vi "TDMS delete channel.vi"(8 "error in (no error)":errorcluster, 9 "Channels":string[](array[string]), 10 "group name":string="Untitled", 11 "file path":path) -> (0 "error out":errorcluster, 1 "Deleted channels":string[](array[string]), 3 "file path out":path)   [LabVIEW 2016]
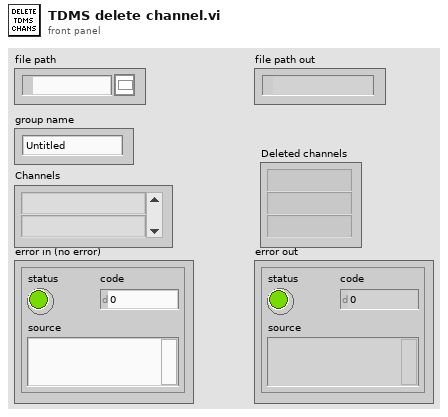
[diagram p1: front panel]
types:
  T1 = enum16{"open", "open or create", "create or replace", "create", "open (read-only)"}
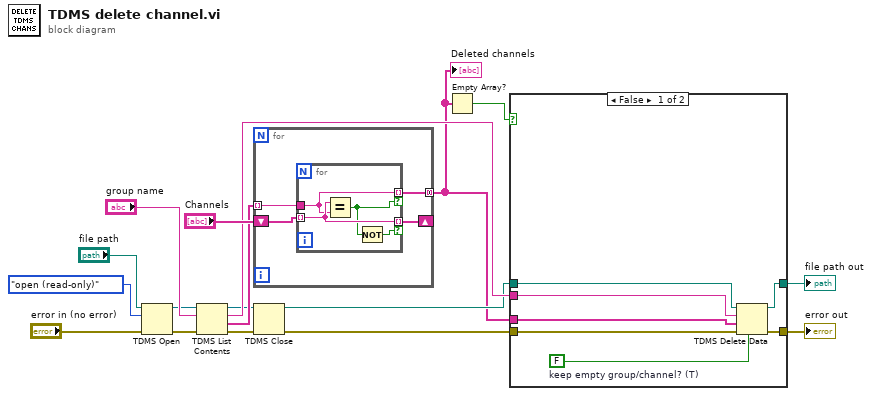
[diagram p0: block diagram]
diagram:
  n1 = TDMS Open(8:"error in (no error)", 10:T1."open (read-only)" ("operation (0:open)"), 11:"file path") -> (0:w13:errorcluster, 3:w16:refnum<k34>)  [unwired: 4 in]
  n2 = TDMS List Contents(4:w13, 6:"group name", 7:w16) -> (0:w9:errorcluster, 1:w11:string[], 2:w10:string, 3:w8:refnum<k34>)
  n3 = for {
    tunnel: w11 -> [w20] mode=indexing
    shift-right: [w19] -> _
    shift-left: "Channels" -> [w21]
    tunnel: [w18] -> w2 mode=concatenating
    n4 = for {
      tunnel: w21 -> [w25] mode=indexing
      tunnel: w20 -> [w23]
      tunnel: [w25] -> w19 mode=indexing if=w24
      tunnel: [w23] -> w18 mode=indexing if=w22
      n5 = Equal?(x=w25, y=w23) -> (x = y?=w22:bool)
      n6 = Not(x=w22) -> (.not. x?=w24:bool)
    }
  }
  "Deleted channels" <- w2
  n7 = TDMS Close(8:w9, 11:w8) -> (0:w5:errorcluster, 3:w6:path)
  n8 = Empty Array?(array=w2) -> (empty?=w1:bool)
  n9 = case shown="False" w1 {
    tunnel: w2 -> [w32 _]
    tunnel: w10 -> [w31 _]
    tunnel: w6 -> [w30 w33]
    tunnel: w5 -> [w29 w34]
    tunnel: [w28 w33] -> w4
    tunnel: [w26 w34] -> w3
    frame False {
      w27 = FALSE  # keep empty group/channel? (T)
      n10 = TDMS Delete Data(6:w27, 8:w29, 9:w32, 10:w31, 11:w30) -> (0:w26:errorcluster, 3:w28:path)  [unwired: 2 in]
    }
    frame True {
    }
  }
  "file path out" <- w4
  "error out" <- w3
